vi "Process Exit Code not Zero--error.vi"(11 "Exit Code":i32) -> (0 "error out":errorcluster)   [LabVIEW 2025]
doc: "Indicates that the executed process terminated with an exit code other than zero."
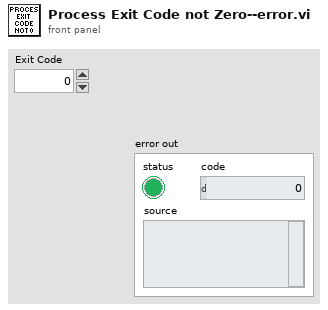
[diagram p1: front panel]
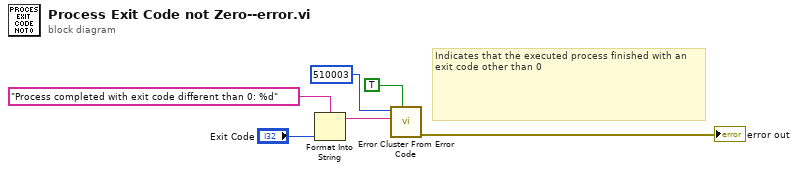
[diagram p0: block diagram]
diagram:
  # "Indicates that the executed process finished with an exit code other than 0"
  n1 = Format Into String(format string="Process completed with exit code different than 0: %d" ("error message (\"\")"), "Exit Code") -> (resulting string=w1:string)  [unwired: 2 in, 1 out]
  n2 = call <vilib>:"Error Cluster From Error Code.vi"("show call chain? (False)"=TRUE, "error message (\"\")"=w1, "error code (0)"=510003) -> ("error out"=→"error out":errorcluster)  [unwired: 6 in]
